vi "Write minutesArc.vi"(8 "error in (no error)":errorcluster, 10 "minutesArc":dbl[unit] min=0.0 max=0.017453292519943295, 11 "Declination in":refnum<class "Declination.lvclass">) -> (0 "error out":errorcluster, 3 "Declination out":refnum<class "Declination.lvclass">)   [LabVIEW 2022 SP3, in "TCSDataDefinitions.lvlib" / "TCSCommand.lvlib" / "TargetConfiguration.lvlib" / "Target.lvlib" / "FixedTarget.lvlib" / "Declination.lvclass"]
uses:
  Declination.lvclass
  Declination.lvclass/Declination.ctl
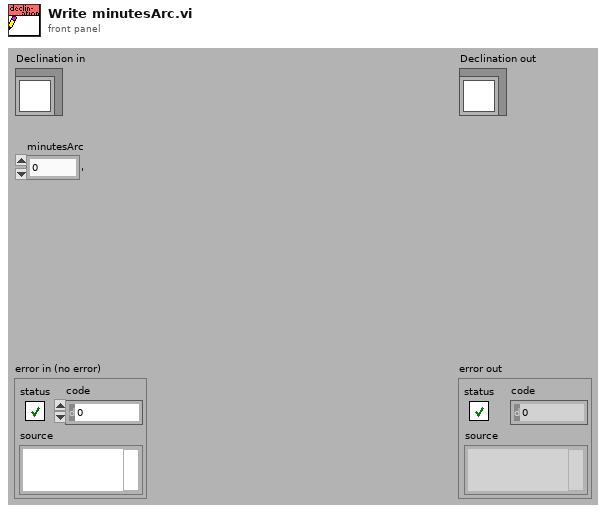
[diagram p1: front panel]
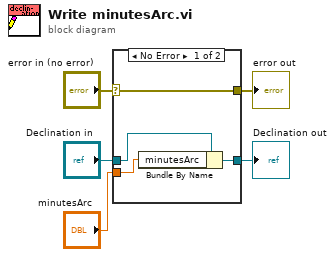
[diagram p0: block diagram]
diagram:
  n1 = case shown="No Error" "error in (no error)" {
    selector: "error in (no error)" -> [w9 w10]
    tunnel: [w9 w10] -> w4
    tunnel: [w7 w11] -> w2
    tunnel: "Declination in" -> [w8 w11]
    tunnel: "minutesArc" -> [w6 _]
    frame No Error {
      n2 = Bundle By Name(cluster=w8, "minutesArc"=w6) -> (w7:refnum<class "Declination.lvclass">)
    }
    frame Error {
    }
  }
  "error out" <- w4
  "Declination out" <- w2
